vi "Calculate Channel Resistance V2.vi"(7 "Scale":i32, 8 "error in (no error)":errorcluster, 9 "ChanSpanOffset":i32, 10 "ChanZeroOffset":i32, 11 "ChanValue":i32) -> (0 "error out":errorcluster, 3 "Channel Ohms Result":dbl)   [LabVIEW 2015]
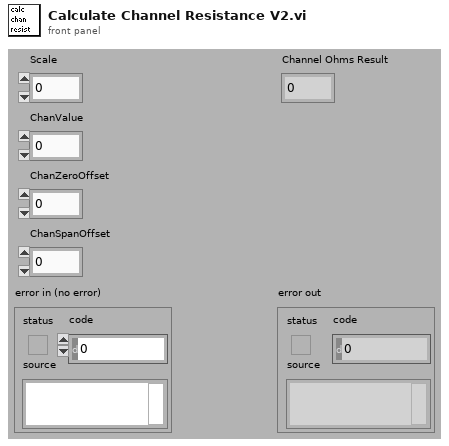
[diagram p1: front panel]
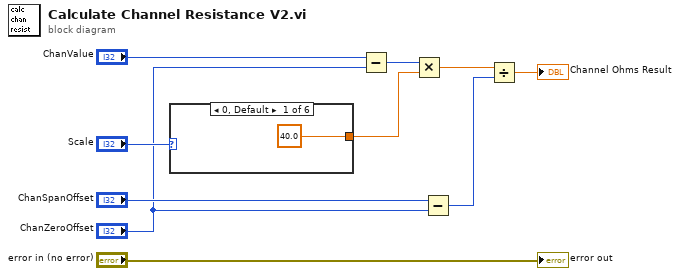
[diagram p0: block diagram]
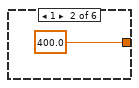
[diagram p2: hidden frame]
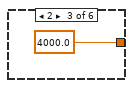
[diagram p3: hidden frame]
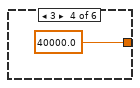
[diagram p4: hidden frame]
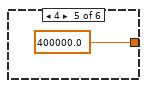
[diagram p5: hidden frame]
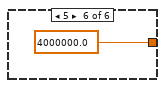
[diagram p6: hidden frame]
diagram:
  n1 = case shown="0, Default" "Scale" {
    tunnel: [40.0 ("Scale") 400.0 ("Scale") 4000.0 ("Scale") 40000.0 ("Scale") 400000.0 ("Scale") 4000000.0 ("Scale")] -> w1
    frame 0, Default {
    }
    frame 1 {
    }
    frame 2 {
    }
    frame 3 {
    }
    frame 4 {
    }
    frame 5 {
    }
  }
  n2 = Subtract(x="ChanValue", y="ChanZeroOffset") -> (x-y=w2:i32)
  n3 = Multiply(x=w2, y=w1) -> (x*y=w5:dbl)
  n4 = Subtract(x="ChanSpanOffset", y="ChanZeroOffset") -> (x-y=w7:i32)
  n5 = Divide(x=w5, y=w7) -> (x/y=→"Channel Ohms Result":dbl)
  "error out" <- "error in (no error)"
